vi "Windspeed Warnings.vi"(8 "Error In":errorcluster, 9 "Weather Data In":T1={"Current Temperature"=0.0, "Max Temperature"=0.0, "Min Temperature"=0.0, "Temperature Warning Text"="No Warning", "Temperatur Warning?"=FALSE, "Units"=enum."Fahrenheit", "Current Windspeed"=0.0, "Max Windspeed"=0.0, "Windspeed Warning?"=FALSE, "Windspeed Warning Text"="No Warning"}) -> (0 "Error Out":errorcluster, 1 "Weather Data Out":T1={"Current Temperature"=0.0, "Max Temperature"=0.0, "Min Temperature"=0.0, "Temperature Warning Text"="No Warning", "Temperatur Warning?"=FALSE, "Units"=enum."Fahrenheit", "Current Windspeed"=0.0, "Max Windspeed"=0.0, "Windspeed Warning?"=FALSE, "Windspeed Warning Text"="No Warning"})   [LabVIEW 2015]
uses:
  Control 1.ctl
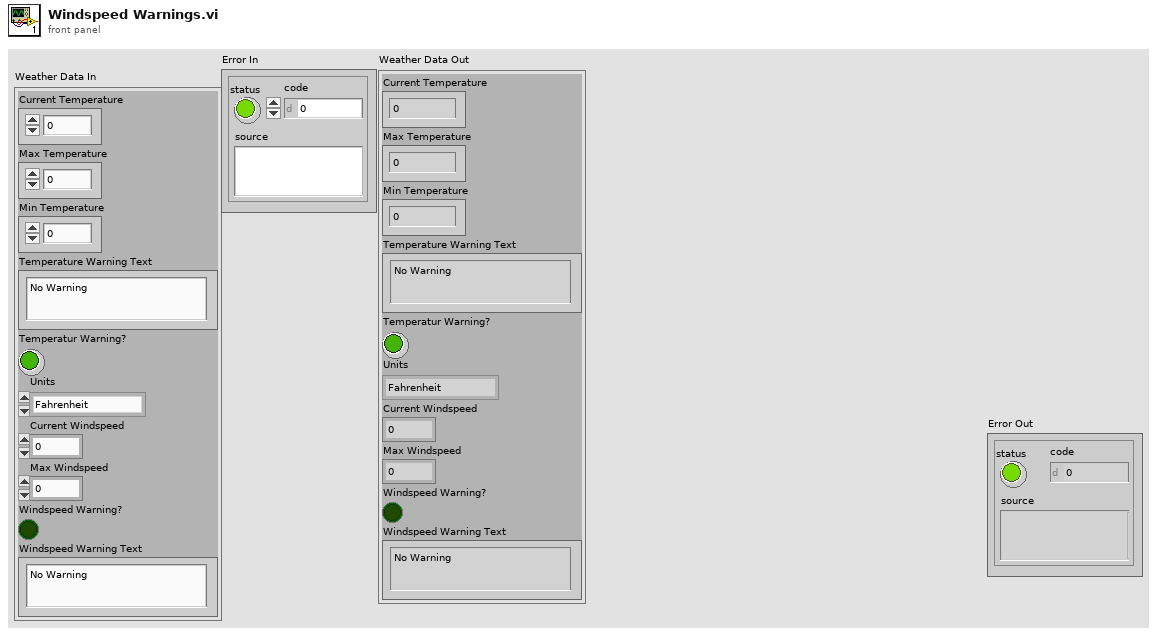
[diagram p1: front panel]
types:
  T1 = typedef "Control 1.ctl" = cluster{"Current Temperature":dbl, "Max Temperature":dbl, "Min Temperature":dbl, "Temperature Warning Text":string, "Temperatur Warning?":bool, "Units":enum16{"Fahrenheit", "Celsius"}, "Current Windspeed":dbl, "Max Windspeed":dbl, "Windspeed Warning?":bool, "Windspeed Warning Text":string}
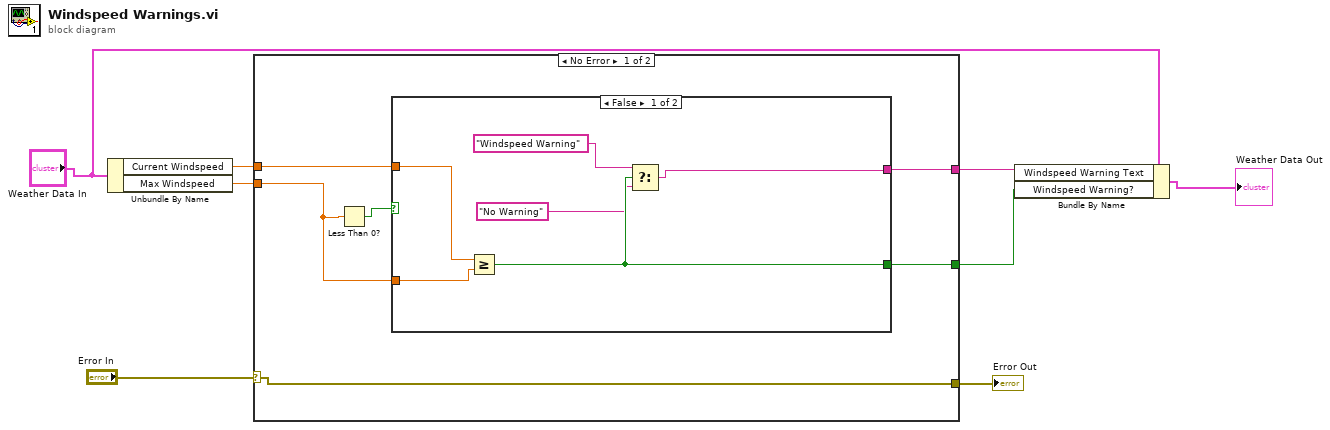
[diagram p0: block diagram]
diagram:
  n1 = Unbundle By Name("Weather Data In") -> ("Current Windspeed"=w6:dbl, "Max Windspeed"=w5:dbl)
  n2 = case shown="No Error" "Error In" {
    selector: "Error In" -> [w14 _]
    tunnel: [w14 _] -> w7
    tunnel: w6 -> [w13 _]
    tunnel: w5 -> [w12 _]
    tunnel: [w10 _] -> w4
    tunnel: [w9 _] -> w2
    frame No Error {
      n3 = Less Than 0?(x=w12) -> (x < 0?=w11:bool)
      n4 = case shown="False" w11 {
        tunnel: w13 -> [w20 _]
        tunnel: w12 -> [w19 _]
        tunnel: [w18 _] -> w10
        tunnel: [w17 _] -> w9
        frame False {
          n5 = Greater Or Equal?(x=w20, y=w19) -> (x >= y?=w18:bool)
          n6 = Select(t="Windspeed Warning", s=w18, f="No Warning") -> (s? t:f=w17:string)
        }
        frame True {
        }
      }
    }
    frame Error {
    }
  }
  "Error Out" <- w7
  n7 = Bundle By Name(cluster="Weather Data In", "Windspeed Warning Text"=w2, "Windspeed Warning?"=w4) -> (→"Weather Data Out":T1)
